vi "AFT Update Coefficients.vi"   [LabVIEW 2017, in "NI_AdaptiveFilter.lvlib"]
doc: "Updates the coefficients of an adaptive filter point by point. Use this VI with the AFT Filter Signal VI to update the coefficients of an adaptive filter. You must use the least mean squares (LMS) or recursive least squares (RLS) algorithms to create the adaptive filter. Wire data to the <B>e(n)</B> input to determine the polymorphic instance to use or manually select the instance. The data type of the adaptive filter that you wire to the <B>adaptive filter in</B> input must match the instance of the AFT Update Coefficients VI."
uses:
  <vilib>/addons/Adaptive Filters/NI_AdaptiveFilter.lvlib
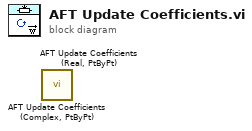
[diagram p0: block diagram]
diagram:
  n1 = call <vilib>:"AFT Update Coefficients (Complex, PtByPt).vi"() -> ()  [unwired: 10 in, 2 out]
  n2 = call <vilib>:"AFT Update Coefficients (Real, PtByPt).vi"() -> ()  [unwired: 10 in, 2 out]
